vi "Initialize.vi"(8 "error in":errorcluster, 10 "InstanceName":string, 11 "Cycler Cluster - 24 Channel.lvclass":refnum<class "Cycler Cluster - 24 Channel.lvclass">) -> (0 "error out":errorcluster, 3 "output cluster":refnum<class "Cycler Cluster - 24 Channel.lvclass">)   [LabVIEW 2023, in "Cycler Cluster - 24 Channel.lvclass"]
uses:
  Cycler Cluster - 24 Channel.lvclass
  Cycler Cluster - 24 Channel.lvclass/Cycler Cluster - 24 Channel.ctl
  7d45be24-9a40-4f36-b3d1-14bc4134107c.vi
  1abf7531-339f-4e14-8fbe-02c4e44e8943.vi
  da48c8f8-b897-4dcf-9451-5b341042a248.vi
  f0f9fcd1-ad99-4552-afb1-31be6853704b.vi
  7d45be24-9a40-4f36-b3d1-14bc4134107c.vi/4bc1c15b-36ab-481f-b8dd-c64075ce723a.vi
  1abf7531-339f-4e14-8fbe-02c4e44e8943.vi/4bc1c15b-36ab-481f-b8dd-c64075ce723a.vi
  da48c8f8-b897-4dcf-9451-5b341042a248.vi/4bc1c15b-36ab-481f-b8dd-c64075ce723a.vi
  f0f9fcd1-ad99-4552-afb1-31be6853704b.vi/4bc1c15b-36ab-481f-b8dd-c64075ce723a.vi
  <vilib>/ADAS Replay HIL/Channels/Tag Wrapper/Polymorphic/Open Producer Tag (Cluster).vi
  <vilib>/ADAS Replay HIL/AdasHilServices/AdasHilServices Fill In Error Info Ex.vi
  <vilib>/ADAS Replay HIL/Channels/Tag Wrapper/Polymorphic/Open Consumer Tag (Cluster).vi
  Utilities/Utilities.lvlib
  <vilib>/ADAS Replay HIL/Channels/Tag Wrapper/Tag Wrapper.lvlib
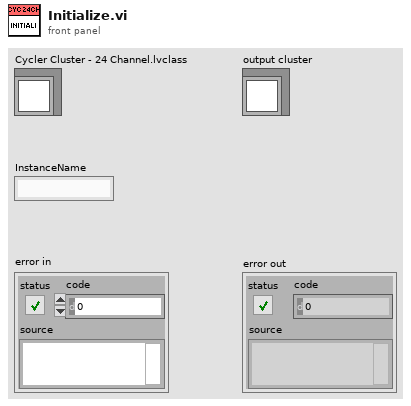
[diagram p1: front panel]
types:
  T1 = cluster{"ErrorAcknowledge.ch01.ACT":bool, "OutputEnable.ch01.ACT":bool, "ControlMode.ch01.CTL":u16, "Voltage.ch01.SP":dbl, "VoltageMIN.ch01.SP":dbl, "VoltageMAX.ch01.SP":dbl, "VoltageGrad.ch01.SP":dbl, "Current.ch01.SP":dbl, "CurrentMIN.ch01.SP":dbl, "CurrentMAX.ch01.SP":dbl, "CurrentGrad.ch01.SP":dbl, "Power.ch01.SP":dbl, "Power.ch01.SP":dbl, "Power.ch01.SP":dbl, "PowerGrad.ch01.SP":dbl, "ParameterSet.ch01.CTL":i32}
  T2 = cluster{"Error.ch01.STS":i32, "OutputEnable.ch01.STS":i32, "ControlMode.ch01.STS":u16, "Voltage.ch01.AV":dbl, "Current.ch01.AV":dbl, "Power.ch01.AV":dbl, "VoltageNominal.ch01.AV":dbl, "CurrentNominal.ch01.AV":dbl, "PowerNominal.ch01.AV":dbl, "ParameterSet.ch01.STS":i32}
  T3 = cluster{"ErrorAcknowledge.ch02.ACT":bool, "OutputEnable.ch02.ACT":bool, "ControlMode.ch02.CTL":u16, "Voltage.ch02.SP":dbl, "VoltageMIN.ch02.SP":dbl, "VoltageMAX.ch02.SP":dbl, "VoltageGrad.ch02.SP":dbl, "Current.ch02.SP":dbl, "CurrentMIN.ch02.SP":dbl, "CurrentMAX.ch02.SP":dbl, "CurrentGrad.ch02.SP":dbl, "Power.ch02.SP":dbl, "PowerMIN.ch02.SP":dbl, "PowerMAX.ch02.SP":dbl, "PowerGrad.ch02.SP":dbl, "ParameterSet.ch02.CTL":i32}
  T4 = cluster{"Error.ch02.STS":i32, "OutputEnable.ch02.STS":i32, "ControlMode.ch02.STS":u16, "Voltage.ch02.AV":dbl, "Current.ch02.AV":dbl, "Power.ch02.AV":dbl, "VoltageNominal.ch02.AV":dbl, "CurrentNominal.ch02.AV":dbl, "PowerNominal.ch02.AV":dbl, "ParameterSet.ch02.STS":i32}
  T5 = cluster{"ErrorAcknowledge.ch03.ACT":bool, "OutputEnable.ch03.ACT":bool, "ControlMode.ch03.CTL":u16, "Voltage.ch03.SP":dbl, "VoltageMIN.ch03.SP":dbl, "VoltageMAX.ch03.SP":dbl, "VoltageGrad.ch03.SP":dbl, "Current.ch03.SP":dbl, "CurrentMIN.ch03.SP":dbl, "CurrentMAX.ch03.SP":dbl, "CurrentGrad.ch03.SP":dbl, "Power.ch03.SP":dbl, "PowerMIN.ch03.SP":dbl, "PowerMAX.ch03.SP":dbl, "PowerGrad.ch03.SP":dbl, "ParameterSet.ch03.CTL":i32}
  T6 = cluster{"Error.ch03.STS":i32, "OutputEnable.ch03.STS":i32, "ControlMode.ch03.STS":u16, "Voltage.ch03.AV":dbl, "Current.ch03.AV":dbl, "Power.ch03.AV":dbl, "VoltageNominal.ch03.AV":dbl, "CurrentNominal.ch03.AV":dbl, "PowerNominal.ch03.AV":dbl, "ParameterSet.ch03.STS":i32}
  T7 = cluster{"ErrorAcknowledge.ch04.ACT":bool, "OutputEnable.ch04.ACT":bool, "ControlMode.ch04.CTL":u16, "Voltage.ch04.SP":dbl, "VoltageMIN.ch04.SP":dbl, "VoltageMAX.ch04.SP":dbl, "VoltageGrad.ch04.SP":dbl, "Current.ch04.SP":dbl, "CurrentMIN.ch04.SP":dbl, "CurrentMAX.ch04.SP":dbl, "CurrentGrad.ch04.SP":dbl, "Power.ch04.SP":dbl, "PowerMIN.ch04.SP":dbl, "PowerMAX.ch04.SP":dbl, "PowerGrad.ch04.SP":dbl, "ParameterSet.ch04.CTL":i32}
  T8 = cluster{"Error.ch04.STS":i32, "OutputEnable.ch04.STS":i32, "ControlMode.ch04.STS":u16, "Voltage.ch04.AV":dbl, "Current.ch04.AV":dbl, "Power.ch04.AV":dbl, "VoltageNominal.ch04.AV":dbl, "CurrentNominal.ch04.AV":dbl, "PowerNominal.ch04.AV":dbl, "ParameterSet.ch04.STS":i32}
  T9 = cluster{"ErrorAcknowledge.ch05.ACT":bool, "OutputEnable.ch05.ACT":bool, "ControlMode.ch05.CTL":u16, "Voltage.ch05.SP":dbl, "VoltageMIN.ch05.SP":dbl, "VoltageMAX.ch05.SP":dbl, "VoltageGrad.ch05.SP":dbl, "Current.ch05.SP":dbl, "CurrentMIN.ch05.SP":dbl, "CurrentMAX.ch05.SP":dbl, "CurrentGrad.ch05.SP":dbl, "Power.ch05.SP":dbl, "PowerMIN.ch05.SP":dbl, "PowerMAX.ch05.SP":dbl, "PowerGrad.ch05.SP":dbl, "ParameterSet.ch05.CTL":i32}
  T10 = cluster{"Error.ch05.STS":i32, "OutputEnable.ch05.STS":i32, "ControlMode.ch05.STS":u16, "Voltage.ch05.AV":dbl, "Current.ch05.AV":dbl, "Power.ch05.AV":dbl, "VoltageNominal.ch05.AV":dbl, "CurrentNominal.ch05.AV":dbl, "PowerNominal.ch05.AV":dbl, "ParameterSet.ch05.STS":i32}
  T11 = cluster{"ErrorAcknowledge.ch06.ACT":bool, "OutputEnable.ch06.ACT":bool, "ControlMode.ch06.CTL":u16, "Voltage.ch06.SP":dbl, "VoltageMIN.ch06.SP":dbl, "VoltageMAX.ch06.SP":dbl, "VoltageGrad.ch06.SP":dbl, "Current.ch06.SP":dbl, "CurrentMIN.ch06.SP":dbl, "CurrentMAX.ch06.SP":dbl, "CurrentGrad.ch06.SP":dbl, "Power.ch06.SP":dbl, "PowerMIN.ch06.SP":dbl, "PowerMAX.ch06.SP":dbl, "PowerGrad.ch06.SP":dbl, "ParameterSet.ch06.CTL":i32}
  T12 = cluster{"Error.ch06.STS":i32, "OutputEnable.ch06.STS":i32, "ControlMode.ch06.STS":u16, "Voltage.ch06.AV":dbl, "Current.ch06.AV":dbl, "Power.ch06.AV":dbl, "VoltageNominal.ch06.AV":dbl, "CurrentNominal.ch06.AV":dbl, "PowerNominal.ch06.AV":dbl, "ParameterSet.ch06.STS":i32}
  T13 = cluster{"ErrorAcknowledge.ch07.ACT":bool, "OutputEnable.ch07.ACT":bool, "ControlMode.ch07.CTL":u16, "Voltage.ch07.SP":dbl, "VoltageMIN.ch07.SP":dbl, "VoltageMAX.ch07.SP":dbl, "VoltageGrad.ch07.SP":dbl, "Current.ch07.SP":dbl, "CurrentMIN.ch07.SP":dbl, "CurrentMAX.ch07.SP":dbl, "CurrentGrad.ch07.SP":dbl, "Power.ch07.SP":dbl, "PowerMIN.ch07.SP":dbl, "PowerMAX.ch07.SP":dbl, "PowerGrad.ch07.SP":dbl, "ParameterSet.ch07.CTL":i32}
  T14 = cluster{"Error.ch07.STS":i32, "OutputEnable.ch07.STS":i32, "ControlMode.ch07.STS":u16, "Voltage.ch07.AV":dbl, "Current.ch07.AV":dbl, "Power.ch07.AV":dbl, "VoltageNominal.ch07.AV":dbl, "CurrentNominal.ch07.AV":dbl, "PowerNominal.ch07.AV":dbl, "ParameterSet.ch07.STS":i32}
  T15 = cluster{"ErrorAcknowledge.ch08.ACT":bool, "OutputEnable.ch08.ACT":bool, "ControlMode.ch08.CTL":u16, "Voltage.ch08.SP":dbl, "VoltageMIN.ch08.SP":dbl, "VoltageMAX.ch08.SP":dbl, "VoltageGrad.ch08.SP":dbl, "Current.ch08.SP":dbl, "CurrentMIN.ch08.SP":dbl, "CurrentMAX.ch08.SP":dbl, "CurrentGrad.ch08.SP":dbl, "Power.ch08.SP":dbl, "PowerMIN.ch08.SP":dbl, "PowerMAX.ch08.SP":dbl, "PowerGrad.ch08.SP":dbl, "ParameterSet.ch08.CTL":i32}
  T16 = cluster{"Error.ch08.STS":i32, "OutputEnable.ch08.STS":i32, "ControlMode.ch08.STS":u16, "Voltage.ch08.AV":dbl, "Current.ch08.AV":dbl, "Power.ch08.AV":dbl, "VoltageNominal.ch08.AV":dbl, "CurrentNominal.ch08.AV":dbl, "PowerNominal.ch08.AV":dbl, "ParameterSet.ch08.STS":i32}
  T17 = cluster{"ErrorAcknowledge.ch09.ACT":bool, "OutputEnable.ch09.ACT":bool, "ControlMode.ch09.CTL":u16, "Voltage.ch09.SP":dbl, "VoltageMIN.ch09.SP":dbl, "VoltageMAX.ch09.SP":dbl, "VoltageGrad.ch09.SP":dbl, "Current.ch09.SP":dbl, "CurrentMIN.ch09.SP":dbl, "CurrentMAX.ch09.SP":dbl, "CurrentGrad.ch09.SP":dbl, "Power.ch09.SP":dbl, "PowerMIN.ch09.SP":dbl, "PowerMAX.ch09.SP":dbl, "PowerGrad.ch09.SP":dbl, "ParameterSet.ch09.CTL":i32}
  T18 = cluster{"Error.ch09.STS":i32, "OutputEnable.ch09.STS":i32, "ControlMode.ch09.STS":u16, "Voltage.ch09.AV":dbl, "Current.ch09.AV":dbl, "Power.ch09.AV":dbl, "VoltageNominal.ch09.AV":dbl, "CurrentNominal.ch09.AV":dbl, "PowerNominal.ch09.AV":dbl, "ParameterSet.ch09.STS":i32}
  T19 = cluster{"ErrorAcknowledge.ch10.ACT":bool, "OutputEnable.ch10.ACT":bool, "ControlMode.ch10.CTL":u16, "Voltage.ch10.SP":dbl, "VoltageMIN.ch10.SP":dbl, "VoltageMAX.ch10.SP":dbl, "VoltageGrad.ch10.SP":dbl, "Current.ch10.SP":dbl, "CurrentMIN.ch10.SP":dbl, "CurrentMAX.ch10.SP":dbl, "CurrentGrad.ch10.SP":dbl, "Power.ch10.SP":dbl, "PowerMIN.ch10.SP":dbl, "PowerMAX.ch10.SP":dbl, "PowerGrad.ch10.SP":dbl, "ParameterSet.ch10.CTL":i32}
  T20 = cluster{"Error.ch10.STS":i32, "OutputEnable.ch10.STS":i32, "ControlMode.ch10.STS":u16, "Voltage.ch10.AV":dbl, "Current.ch10.AV":dbl, "Power.ch10.AV":dbl, "VoltageNominal.ch10.AV":dbl, "CurrentNominal.ch10.AV":dbl, "PowerNominal.ch10.AV":dbl, "ParameterSet.ch10.STS":i32}
  T21 = cluster{"ErrorAcknowledge.ch11.ACT":bool, "OutputEnable.ch11.ACT":bool, "ControlMode.ch11.CTL":u16, "Voltage.ch11.SP":dbl, "VoltageMIN.ch11.SP":dbl, "VoltageMAX.ch11.SP":dbl, "VoltageGrad.ch11.SP":dbl, "Current.ch11.SP":dbl, "CurrentMIN.ch11.SP":dbl, "CurrentMAX.ch11.SP":dbl, "CurrentGrad.ch11.SP":dbl, "Power.ch11.SP":dbl, "PowerMIN.ch11.SP":dbl, "PowerMAX.ch11.SP":dbl, "PowerGrad.ch11.SP":dbl, "ParameterSet.ch11.CTL":i32}
  T22 = cluster{"Error.ch11.STS":i32, "OutputEnable.ch11.STS":i32, "ControlMode.ch11.STS":u16, "Voltage.ch11.AV":dbl, "Current.ch11.AV":dbl, "Power.ch11.AV":dbl, "VoltageNominal.ch11.AV":dbl, "CurrentNominal.ch11.AV":dbl, "PowerNominal.ch11.AV":dbl, "ParameterSet.ch11.STS":i32}
  T23 = cluster{"ErrorAcknowledge.ch12.ACT":bool, "OutputEnable.ch12.ACT":bool, "ControlMode.ch12.CTL":u16, "Voltage.ch12.SP":dbl, "VoltageMIN.ch12.SP":dbl, "VoltageMAX.ch12.SP":dbl, "VoltageGrad.ch12.SP":dbl, "Current.ch12.SP":dbl, "CurrentMIN.ch12.SP":dbl, "CurrentMAX.ch12.SP":dbl, "CurrentGrad.ch12.SP":dbl, "Power.ch12.SP":dbl, "PowerMIN.ch12.SP":dbl, "PowerMAX.ch12.SP":dbl, "PowerGrad.ch12.SP":dbl, "ParameterSet.ch12.CTL":i32}
  T24 = cluster{"Error.ch12.STS":i32, "OutputEnable.ch12.STS":i32, "ControlMode.ch12.STS":u16, "Voltage.ch12.AV":dbl, "Current.ch12.AV":dbl, "Power.ch12.AV":dbl, "VoltageNominal.ch12.AV":dbl, "CurrentNominal.ch12.AV":dbl, "PowerNominal.ch12.AV":dbl, "ParameterSet.ch12.STS":i32}
  T25 = cluster{"ErrorAcknowledge.ch13.ACT":bool, "OutputEnable.ch13.ACT":bool, "ControlMode.ch13.CTL":u16, "Voltage.ch13.SP":dbl, "VoltageMIN.ch13.SP":dbl, "VoltageMAX.ch13.SP":dbl, "VoltageGrad.ch13.SP":dbl, "Current.ch13.SP":dbl, "CurrentMIN.ch13.SP":dbl, "CurrentMAX.ch13.SP":dbl, "CurrentGrad.ch13.SP":dbl, "Power.ch13.SP":dbl, "PowerMIN.ch13.SP":dbl, "PowerMAX.ch13.SP":dbl, "PowerGrad.ch13.SP":dbl, "ParameterSet.ch13.CTL":i32}
  T26 = cluster{"Error.ch13.STS":i32, "OutputEnable.ch13.STS":i32, "ControlMode.ch13.STS":u16, "Voltage.ch13.AV":dbl, "Current.ch13.AV":dbl, "Power.ch13.AV":dbl, "VoltageNominal.ch13.AV":dbl, "CurrentNominal.ch13.AV":dbl, "PowerNominal.ch13.AV":dbl, "ParameterSet.ch13.STS":i32}
  T27 = cluster{"ErrorAcknowledge.ch14.ACT":bool, "OutputEnable.ch14.ACT":bool, "ControlMode.ch14.CTL":u16, "Voltage.ch14.SP":dbl, "VoltageMIN.ch14.SP":dbl, "VoltageMAX.ch14.SP":dbl, "VoltageGrad.ch14.SP":dbl, "Current.ch14.SP":dbl, "CurrentMIN.ch14.SP":dbl, "CurrentMAX.ch14.SP":dbl, "CurrentGrad.ch14.SP":dbl, "Power.ch14.SP":dbl, "PowerMIN.ch14.SP":dbl, "PowerMAX.ch14.SP":dbl, "PowerGrad.ch14.SP":dbl, "ParameterSet.ch14.CTL":i32}
  T28 = cluster{"Error.ch14.STS":i32, "OutputEnable.ch14.STS":i32, "ControlMode.ch14.STS":u16, "Voltage.ch14.AV":dbl, "Current.ch14.AV":dbl, "Power.ch14.AV":dbl, "VoltageNominal.ch14.AV":dbl, "CurrentNominal.ch14.AV":dbl, "PowerNominal.ch14.AV":dbl, "ParameterSet.ch14.STS":i32}
  T29 = cluster{"ErrorAcknowledge.ch15.ACT":bool, "OutputEnable.ch15.ACT":bool, "ControlMode.ch15.CTL":u16, "Voltage.ch15.SP":dbl, "VoltageMIN.ch15.SP":dbl, "VoltageMAX.ch15.SP":dbl, "VoltageGrad.ch15.SP":dbl, "Current.ch15.SP":dbl, "CurrentMIN.ch15.SP":dbl, "CurrentMAX.ch15.SP":dbl, "CurrentGrad.ch15.SP":dbl, "Power.ch15.SP":dbl, "PowerMIN.ch15.SP":dbl, "PowerMAX.ch15.SP":dbl, "PowerGrad.ch15.SP":dbl, "ParameterSet.ch15.CTL":i32}
  T30 = cluster{"Error.ch15.STS":i32, "OutputEnable.ch15.STS":i32, "ControlMode.ch15.STS":u16, "Voltage.ch15.AV":dbl, "Current.ch15.AV":dbl, "Power.ch15.AV":dbl, "VoltageNominal.ch15.AV":dbl, "CurrentNominal.ch15.AV":dbl, "PowerNominal.ch15.AV":dbl, "ParameterSet.ch15.STS":i32}
  T31 = cluster{"ErrorAcknowledge.ch16.ACT":bool, "OutputEnable.ch16.ACT":bool, "ControlMode.ch16.CTL":u16, "Voltage.ch16.SP":dbl, "VoltageMIN.ch16.SP":dbl, "VoltageMAX.ch16.SP":dbl, "VoltageGrad.ch16.SP":dbl, "Current.ch16.SP":dbl, "CurrentMIN.ch16.SP":dbl, "CurrentMAX.ch16.SP":dbl, "CurrentGrad.ch16.SP":dbl, "Power.ch16.SP":dbl, "PowerMIN.ch16.SP":dbl, "PowerMAX.ch16.SP":dbl, "PowerGrad.ch16.SP":dbl, "ParameterSet.ch16.CTL":i32}
  T32 = cluster{"Error.ch16.STS":i32, "OutputEnable.ch16.STS":i32, "ControlMode.ch16.STS":u16, "Voltage.ch16.AV":dbl, "Current.ch16.AV":dbl, "Power.ch16.AV":dbl, "VoltageNominal.ch16.AV":dbl, "CurrentNominal.ch16.AV":dbl, "PowerNominal.ch16.AV":dbl, "ParameterSet.ch16.STS":i32}
  T33 = cluster{"ErrorAcknowledge.ch17.ACT":bool, "OutputEnable.ch17.ACT":bool, "ControlMode.ch17.CTL":u16, "Voltage.ch17.SP":dbl, "VoltageMIN.ch17.SP":dbl, "VoltageMAX.ch17.SP":dbl, "VoltageGrad.ch17.SP":dbl, "Current.ch17.SP":dbl, "CurrentMIN.ch17.SP":dbl, "CurrentMAX.ch17.SP":dbl, "CurrentGrad.ch17.SP":dbl, "Power.ch17.SP":dbl, "PowerMIN.ch17.SP":dbl, "PowerMAX.ch17.SP":dbl, "PowerGrad.ch17.SP":dbl, "ParameterSet.ch17.CTL":i32}
  T34 = cluster{"Error.ch17.STS":i32, "OutputEnable.ch17.STS":i32, "ControlMode.ch17.STS":u16, "Voltage.ch17.AV":dbl, "Current.ch17.AV":dbl, "Power.ch17.AV":dbl, "VoltageNominal.ch17.AV":dbl, "CurrentNominal.ch17.AV":dbl, "PowerNominal.ch17.AV":dbl, "ParameterSet.ch17.STS":i32}
  T35 = cluster{"ErrorAcknowledge.ch18.ACT":bool, "OutputEnable.ch18.ACT":bool, "ControlMode.ch18.CTL":u16, "Voltage.ch18.SP":dbl, "VoltageMIN.ch18.SP":dbl, "VoltageMAX.ch18.SP":dbl, "VoltageGrad.ch18.SP":dbl, "Current.ch18.SP":dbl, "CurrentMIN.ch18.SP":dbl, "CurrentMAX.ch18.SP":dbl, "CurrentGrad.ch18.SP":dbl, "Power.ch18.SP":dbl, "PowerMIN.ch18.SP":dbl, "PowerMAX.ch18.SP":dbl, "PowerGrad.ch18.SP":dbl, "ParameterSet.ch18.CTL":i32}
  T36 = cluster{"Error.ch18.STS":i32, "OutputEnable.ch18.STS":i32, "ControlMode.ch18.STS":u16, "Voltage.ch18.AV":dbl, "Current.ch18.AV":dbl, "Power.ch18.AV":dbl, "VoltageNominal.ch18.AV":dbl, "CurrentNominal.ch18.AV":dbl, "PowerNominal.ch18.AV":dbl, "ParameterSet.ch18.STS":i32}
  T37 = cluster{"ErrorAcknowledge.ch19.ACT":bool, "OutputEnable.ch19.ACT":bool, "ControlMode.ch19.CTL":u16, "Voltage.ch19.SP":dbl, "VoltageMIN.ch19.SP":dbl, "VoltageMAX.ch19.SP":dbl, "VoltageGrad.ch19.SP":dbl, "Current.ch19.SP":dbl, "CurrentMIN.ch19.SP":dbl, "CurrentMAX.ch19.SP":dbl, "CurrentGrad.ch19.SP":dbl, "Power.ch19.SP":dbl, "PowerMIN.ch19.SP":dbl, "PowerMAX.ch19.SP":dbl, "PowerGrad.ch19.SP":dbl, "ParameterSet.ch19.CTL":i32}
  T38 = cluster{"Error.ch19.STS":i32, "OutputEnable.ch19.STS":i32, "ControlMode.ch19.STS":u16, "Voltage.ch19.AV":dbl, "Current.ch19.AV":dbl, "Power.ch19.AV":dbl, "VoltageNominal.ch19.AV":dbl, "CurrentNominal.ch19.AV":dbl, "PowerNominal.ch19.AV":dbl, "ParameterSet.ch19.STS":i32}
  T39 = cluster{"ErrorAcknowledge.ch20.ACT":bool, "OutputEnable.ch20.ACT":bool, "ControlMode.ch20.CTL":u16, "Voltage.ch20.SP":dbl, "VoltageMIN.ch20.SP":dbl, "VoltageMAX.ch20.SP":dbl, "VoltageGrad.ch20.SP":dbl, "Current.ch20.SP":dbl, "CurrentMIN.ch20.SP":dbl, "CurrentMAX.ch20.SP":dbl, "CurrentGrad.ch20.SP":dbl, "Power.ch20.SP":dbl, "PowerMIN.ch20.SP":dbl, "PowerMAX.ch20.SP":dbl, "PowerGrad.ch20.SP":dbl, "ParameterSet.ch20.CTL":i32}
  T40 = cluster{"Error.ch20.STS":i32, "OutputEnable.ch20.STS":i32, "ControlMode.ch20.STS":u16, "Voltage.ch20.AV":dbl, "Current.ch20.AV":dbl, "Power.ch20.AV":dbl, "VoltageNominal.ch20.AV":dbl, "CurrentNominal.ch20.AV":dbl, "PowerNominal.ch20.AV":dbl, "ParameterSet.ch20.STS":i32}
  T41 = cluster{"ErrorAcknowledge.ch21.ACT":bool, "OutputEnable.ch21.ACT":bool, "ControlMode.ch21.CTL":u16, "Voltage.ch21.SP":dbl, "VoltageMIN.ch21.SP":dbl, "VoltageMAX.ch21.SP":dbl, "VoltageGrad.ch21.SP":dbl, "Current.ch21.SP":dbl, "CurrentMIN.ch21.SP":dbl, "CurrentMAX.ch21.SP":dbl, "CurrentGrad.ch21.SP":dbl, "Power.ch21.SP":dbl, "PowerMIN.ch21.SP":dbl, "PowerMAX.ch21.SP":dbl, "PowerGrad.ch21.SP":dbl, "ParameterSet.ch21.CTL":i32}
  T42 = cluster{"Error.ch21.STS":i32, "OutputEnable.ch21.STS":i32, "ControlMode.ch21.STS":u16, "Voltage.ch21.AV":dbl, "Current.ch21.AV":dbl, "Power.ch21.AV":dbl, "VoltageNominal.ch21.AV":dbl, "CurrentNominal.ch21.AV":dbl, "PowerNominal.ch21.AV":dbl, "ParameterSet.ch21.STS":i32}
  T43 = cluster{"ErrorAcknowledge.ch22.ACT":bool, "OutputEnable.ch22.ACT":bool, "ControlMode.ch22.CTL":u16, "Voltage.ch22.SP":dbl, "VoltageMIN.ch22.SP":dbl, "VoltageMAX.ch22.SP":dbl, "VoltageGrad.ch22.SP":dbl, "Current.ch22.SP":dbl, "CurrentMIN.ch22.SP":dbl, "CurrentMAX.ch22.SP":dbl, "CurrentGrad.ch22.SP":dbl, "Power.ch22.SP":dbl, "PowerMIN.ch22.SP":dbl, "PowerMAX.ch22.SP":dbl, "PowerGrad.ch22.SP":dbl, "ParameterSet.ch22.CTL":i32}
  T44 = cluster{"Error.ch22.STS":i32, "OutputEnable.ch22.STS":i32, "ControlMode.ch22.STS":u16, "Voltage.ch22.AV":dbl, "Current.ch22.AV":dbl, "Power.ch22.AV":dbl, "VoltageNominal.ch22.AV":dbl, "CurrentNominal.ch22.AV":dbl, "PowerNominal.ch22.AV":dbl, "ParameterSet.ch22.STS":i32}
  T45 = cluster{"ErrorAcknowledge.ch23.ACT":bool, "OutputEnable.ch23.ACT":bool, "ControlMode.ch23.CTL":u16, "Voltage.ch23.SP":dbl, "VoltageMIN.ch23.SP":dbl, "VoltageMAX.ch23.SP":dbl, "VoltageGrad.ch23.SP":dbl, "Current.ch23.SP":dbl, "CurrentMIN.ch23.SP":dbl, "CurrentMAX.ch23.SP":dbl, "CurrentGrad.ch23.SP":dbl, "Power.ch23.SP":dbl, "PowerMIN.ch23.SP":dbl, "PowerMAX.ch23.SP":dbl, "PowerGrad.ch23.SP":dbl, "ParameterSet.ch23.CTL":i32}
  T46 = cluster{"Error.ch23.STS":i32, "OutputEnable.ch23.STS":i32, "ControlMode.ch23.STS":u16, "Voltage.ch23.AV":dbl, "Current.ch23.AV":dbl, "Power.ch23.AV":dbl, "VoltageNominal.ch23.AV":dbl, "CurrentNominal.ch23.AV":dbl, "PowerNominal.ch23.AV":dbl, "ParameterSet.ch23.STS":i32}
  T47 = cluster{"ErrorAcknowledge.ch24.ACT":bool, "OutputEnable.ch24.ACT":bool, "ControlMode.ch24.CTL":u16, "Voltage.ch24.SP":dbl, "VoltageMIN.ch24.SP":dbl, "VoltageMAX.ch24.SP":dbl, "VoltageGrad.ch24.SP":dbl, "Current.ch24.SP":dbl, "CurrentMIN.ch24.SP":dbl, "CurrentMAX.ch24.SP":dbl, "CurrentGrad.ch24.SP":dbl, "Power.ch24.SP":dbl, "PowerMIN.ch24.SP":dbl, "PowerMAX.ch24.SP":dbl, "PowerGrad.ch24.SP":dbl, "ParameterSet.ch24.CTL":i32}
  T48 = cluster{"Error.ch24.STS":i32, "OutputEnable.ch24.STS":i32, "ControlMode.ch24.STS":u16, "Voltage.ch24.AV":dbl, "Current.ch24.AV":dbl, "Power.ch24.AV":dbl, "VoltageNominal.ch24.AV":dbl, "CurrentNominal.ch24.AV":dbl, "PowerNominal.ch24.AV":dbl, "ParameterSet.ch24.STS":i32}
  T49 = cluster{"ErrorAcknowledge.ch24.ACT":bool, "OutputEnable.ch24.ACT":bool, "ControlMode.ch24.CTL":u16, "Voltage.ch24.SP":dbl, "VoltageMIN.ch24.SP":dbl, "VoltageMAX.ch24.SP":dbl, "VoltageGrad.ch24.SP":dbl, "Current.ch24.SP":dbl, "CurrentMIN.ch24.SP":dbl, "CurrentMAX.ch24.SP":dbl, "CurrentGrad.ch24.SP":dbl, "Power.ch24.SP":dbl, "PowerMIN.ch24.SP":dbl, "PowerMAX.ch24.SP":dbl, "PowerGrad.ch24.SP":dbl, "ParameterSet.ch24.CTL":i32}[]
  T50 = cluster{"Error.ch24.STS":i32, "OutputEnable.ch24.STS":i32, "ControlMode.ch24.STS":u16, "Voltage.ch24.AV":dbl, "Current.ch24.AV":dbl, "Power.ch24.AV":dbl, "VoltageNominal.ch24.AV":dbl, "CurrentNominal.ch24.AV":dbl, "PowerNominal.ch24.AV":dbl, "ParameterSet.ch24.STS":i32}[]
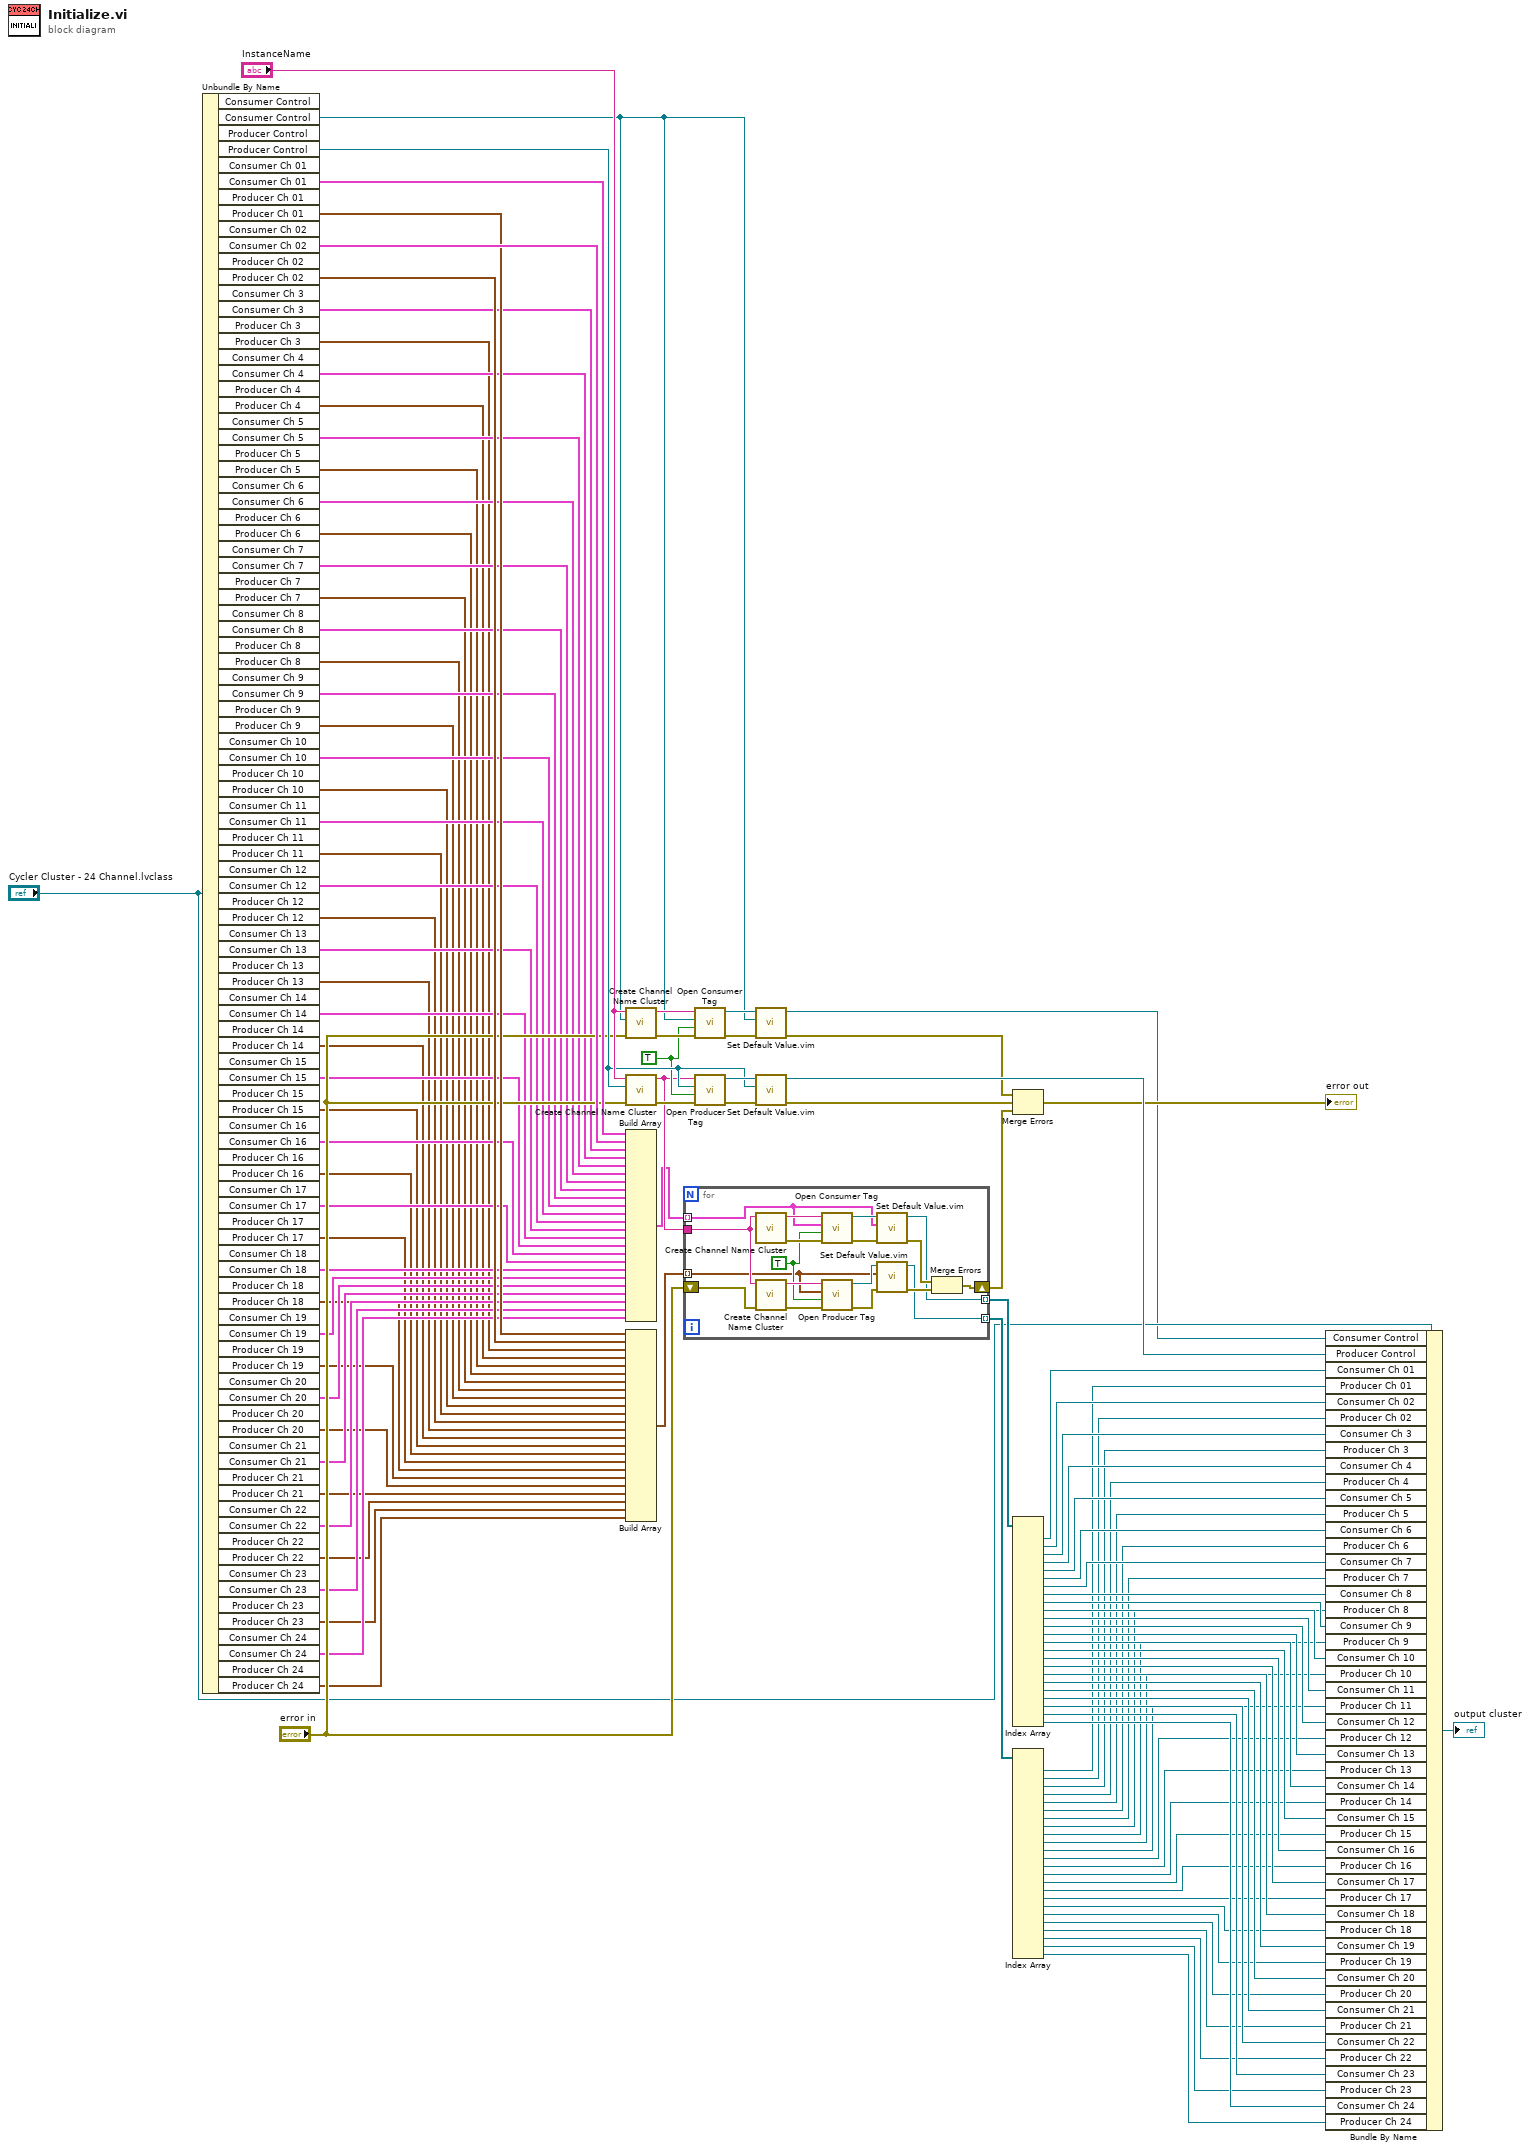
[diagram p0: block diagram]
diagram:
  w104 = TRUE ("Create if not found? (T)")
  n1 = Unbundle By Name("Cycler Cluster - 24 Channel.lvclass") -> ("Consumer Control"=w108:refnum<k21>, "Producer Control"=w107:refnum<k21>, "Consumer Ch 01"=w106:T1, "Producer Ch 01"=w102:T2, "Consumer Ch 02"=w105:T3, "Producer Ch 02"=w101:T4, "Consumer Ch 3"=w94:T5, "Producer Ch 3"=w72:T6, "Consumer Ch 4"=w93:T7, "Producer Ch 4"=w71:T8, "Consumer Ch 5"=w92:T9, "Producer Ch 5"=w70:T10, "Consumer Ch 6"=w91:T11, "Producer Ch 6"=w69:T12, "Consumer Ch 7"=w90:T13, "Producer Ch 7"=w68:T14, "Consumer Ch 8"=w89:T15, "Producer Ch 8"=w67:T16, "Consumer Ch 9"=w88:T17, "Producer Ch 9"=w66:T18, "Consumer Ch 10"=w87:T19, "Producer Ch 10"=w65:T20, "Consumer Ch 11"=w86:T21, "Producer Ch 11"=w64:T22, "Consumer Ch 12"=w85:T23, "Producer Ch 12"=w63:T24, "Consumer Ch 13"=w84:T25, "Producer Ch 13"=w62:T26, "Consumer Ch 14"=w83:T27, "Producer Ch 14"=w61:T28, "Consumer Ch 15"=w82:T29, "Producer Ch 15"=w60:T30, "Consumer Ch 16"=w81:T31, "Producer Ch 16"=w59:T32, "Consumer Ch 17"=w80:T33, "Producer Ch 17"=w58:T34, "Consumer Ch 18"=w79:T35, "Producer Ch 18"=w57:T36, "Consumer Ch 19"=w78:T37, "Producer Ch 19"=w56:T38, "Consumer Ch 20"=w77:T39, "Producer Ch 20"=w55:T40, "Consumer Ch 21"=w76:T41, "Producer Ch 21"=w54:T42, "Consumer Ch 22"=w75:T43, "Producer Ch 22"=w53:T44, "Consumer Ch 23"=w74:T45, "Producer Ch 23"=w52:T46, "Consumer Ch 24"=w73:T47, "Producer Ch 24"=w51:T48)  [unwired: 50 out]
  n2 = call "Create Channel Name Cluster.vi"("error in"="error in", "Cluster"=w108, "Instance Name"="InstanceName") -> ("error out"=w114:errorcluster, "Data Channel Name"=w121:string)  [unwired: 7 in]
  n3 = call "Create Channel Name Cluster.vi"("error in"="error in", "Cluster"=w107, "Instance Name"="InstanceName") -> ("error out"=w115:errorcluster, "Data Channel Name"=w103:string)  [unwired: 7 in]
  n4 = Build Array(w106, w105, w94, w93, w92, w91, w90, w89, w88, w87, w86, w85, w84, w83, w82, w81, w80, w79, w78, w77, w76, w75, w74, w73) -> (w1:T49)
  n5 = Build Array(w102, w101, w72, w71, w70, w69, w68, w67, w66, w65, w64, w63, w62, w61, w60, w59, w58, w57, w56, w55, w54, w53, w52, w51) -> (w100:T50)
  n6 = for {
    tunnel: w103 -> [w130]
    tunnel: w1 -> [w122] mode=indexing
    tunnel: w100 -> [w129] mode=indexing
    shift-right: [w125] -> w98
    shift-left: "error in" -> [w128]
    tunnel: [w124] -> w96 mode=indexing
    tunnel: [w123] -> w28 mode=indexing
    w131 = TRUE ("Create if not found? (T)")
    n7 = call "Create Channel Name Cluster.vi"("Instance Name"=w130) -> ("error out"=w132:errorcluster, "Data Channel Name"=w139:string)  [unwired: 9 in]
    n8 = call "Create Channel Name Cluster.vi"("error in"=w128, "Instance Name"=w130) -> ("error out"=w133:errorcluster, "Data Channel Name"=w138:string)  [unwired: 8 in]
    n9 = call-poly <vilib>:"Open Consumer Tag.vi"("error in"=w132, "Create if not found? (T)"=w131, "Cluster"=w122, "Channel Name"=w139) -> ("error out"=w136:errorcluster, "ADAS HIL Channel"=w137:refnum<k21>)  [unwired: 6 in]
    n10 = call-poly <vilib>:"Open Producer Tag.vi"("error in"=w133, "Create if not found? (T)"=w131, "Cluster"=w129, "Channel Name"=w138) -> ("error out"=w135:errorcluster, "ADAS HIL Channel"=w134:refnum<k21>)  [unwired: 6 in]
    n11 = call "Set Default Value.vim"("error in"=w136, "Data in"=w122, "ADAS HIL Channel in"=w137) -> ("error out"=w126:errorcluster, "ADAS HIL Channel out"=w124:refnum<k21>)  [unwired: 7 in]
    n12 = call "Set Default Value.vim"("error in"=w135, "Data in"=w129, "ADAS HIL Channel in"=w134) -> ("error out"=w127:errorcluster, "ADAS HIL Channel out"=w123:refnum<k21>)  [unwired: 7 in]
    n13 = Merge Errors(w126, w127) -> (w125:errorcluster)
  }
  n14 = call-poly <vilib>:"Open Consumer Tag.vi"("error in"=w114, "Create if not found? (T)"=w104, "Cluster"=w108, "Channel Name"=w121) -> ("error out"=w119:errorcluster, "ADAS HIL Channel"=w120:refnum<k21>)  [unwired: 6 in]
  n15 = call-poly <vilib>:"Open Producer Tag.vi"("error in"=w115, "Create if not found? (T)"=w104, "Cluster"=w107, "Channel Name"=w103) -> ("error out"=w118:errorcluster, "ADAS HIL Channel"=w117:refnum<k21>)  [unwired: 6 in]
  n16 = call "Set Default Value.vim"("error in"=w119, "Data in"=w108, "ADAS HIL Channel in"=w120) -> ("error out"=w113:errorcluster, "ADAS HIL Channel out"=w2:refnum<k21>)  [unwired: 7 in]
  n17 = call "Set Default Value.vim"("error in"=w118, "Data in"=w107, "ADAS HIL Channel in"=w117) -> ("error out"=w112:errorcluster, "ADAS HIL Channel out"=w116:refnum<k21>)  [unwired: 7 in]
  n18 = Merge Errors(w113, w112, w98) -> (→"error out":errorcluster)
  n19 = Index Array(array=w96) -> (element #1=w97:refnum<k21>, element #2=w95:refnum<k21>, element #3=w50:refnum<k21>, element #4=w49:refnum<k21>, element #5=w48:refnum<k21>, element #6=w47:refnum<k21>, element #7=w46:refnum<k21>, element #8=w45:refnum<k21>, element #9=w44:refnum<k21>, element #10=w43:refnum<k21>, element #11=w42:refnum<k21>, element #12=w41:refnum<k21>, element #13=w40:refnum<k21>, element #14=w39:refnum<k21>, element #15=w38:refnum<k21>, element #16=w37:refnum<k21>, element #17=w36:refnum<k21>, element #18=w35:refnum<k21>, element #19=w34:refnum<k21>, element #20=w33:refnum<k21>, element #21=w32:refnum<k21>, element #22=w31:refnum<k21>, element #23=w30:refnum<k21>, element #24=w29:refnum<k21>)  [unwired: 24 in]
  n20 = Index Array(array=w28) -> (element #1=w27:refnum<k21>, element #2=w26:refnum<k21>, element #3=w25:refnum<k21>, element #4=w24:refnum<k21>, element #5=w23:refnum<k21>, element #6=w22:refnum<k21>, element #7=w21:refnum<k21>, element #8=w20:refnum<k21>, element #9=w19:refnum<k21>, element #10=w18:refnum<k21>, element #11=w17:refnum<k21>, element #12=w16:refnum<k21>, element #13=w15:refnum<k21>, element #14=w14:refnum<k21>, element #15=w13:refnum<k21>, element #16=w12:refnum<k21>, element #17=w11:refnum<k21>, element #18=w10:refnum<k21>, element #19=w9:refnum<k21>, element #20=w8:refnum<k21>, element #21=w7:refnum<k21>, element #22=w6:refnum<k21>, element #23=w5:refnum<k21>, element #24=w4:refnum<k21>)  [unwired: 24 in]
  n21 = Bundle By Name(cluster="Cycler Cluster - 24 Channel.lvclass", "Consumer Control"=w2, "Producer Control"=w116, "Consumer Ch 01"=w97, "Producer Ch 01"=w27, "Consumer Ch 02"=w95, "Producer Ch 02"=w26, "Consumer Ch 3"=w50, "Producer Ch 3"=w25, "Consumer Ch 4"=w49, "Producer Ch 4"=w24, "Consumer Ch 5"=w48, "Producer Ch 5"=w23, "Consumer Ch 6"=w47, "Producer Ch 6"=w22, "Consumer Ch 7"=w46, "Producer Ch 7"=w21, "Consumer Ch 8"=w45, "Producer Ch 8"=w20, "Consumer Ch 9"=w44, "Producer Ch 9"=w19, "Consumer Ch 10"=w43, "Producer Ch 10"=w18, "Consumer Ch 11"=w42, "Producer Ch 11"=w17, "Consumer Ch 12"=w41, "Producer Ch 12"=w16, "Consumer Ch 13"=w40, "Producer Ch 13"=w15, "Consumer Ch 14"=w39, "Producer Ch 14"=w14, "Consumer Ch 15"=w38, "Producer Ch 15"=w13, "Consumer Ch 16"=w37, "Producer Ch 16"=w12, "Consumer Ch 17"=w36, "Producer Ch 17"=w11, "Consumer Ch 18"=w35, "Producer Ch 18"=w10, "Consumer Ch 19"=w34, "Producer Ch 19"=w9, "Consumer Ch 20"=w33, "Producer Ch 20"=w8, "Consumer Ch 21"=w32, "Producer Ch 21"=w7, "Consumer Ch 22"=w31, "Producer Ch 22"=w6, "Consumer Ch 23"=w30, "Producer Ch 23"=w5, "Consumer Ch 24"=w29, "Producer Ch 24"=w4) -> (→"output cluster":refnum<class "Cycler Cluster - 24 Channel.lvclass">)
